vi "LuaVIEW Push (flat data).vi"(0 "flat data":string, 2 "type descriptor":i16[](array[numeric]) format="%x", 5 "LuaVIEW reference in":T1, 7 "include cluster order (false)":bool, 11 "error in (no error)":errorcluster) -> (6 "LuaVIEW reference out":T1, 15 "error out":errorcluster)   [LabVIEW 2013]
doc: "Pushes a Lua-data item onto the stack after translating it from flat LabVIEW data. The most important use for this VI is to transfer compound data from LabVIEW (a cluster or array) to Lua (a table). To perform the translation, this function requires the type descriptor of the LabVIEW type/cluster/array that specifies how the translation is to take place. The translation is recursive and thus handles nested clusters and arrays. If no translation is possible, e.g. because cluster elements are not named, an error is returned. The LuaVIEW manual details which translations are supported. This VI is part of a polymorphic set that supports pushing various data types. To change the type being pushed, pop up on this VI's diagram icon and use the \"Select Type\" sub menu."
uses:
  typedefs/t_LuaVIEW Reference.ctl
  typedefs/et_LuaVIEW CIN Actions.ctl
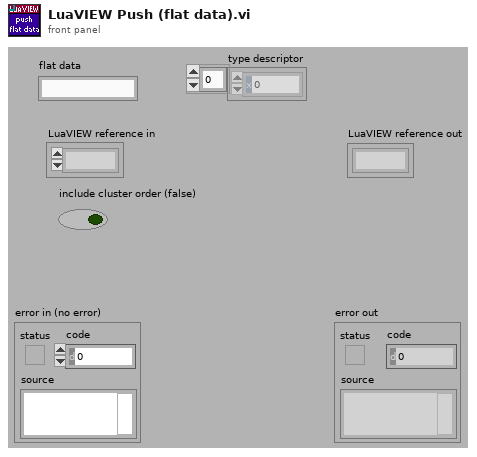
[diagram p1: front panel]
types:
  T1 = typedef "t_LuaVIEW Reference.ctl" = refnum<k1>
  T2 = typedef "et_LuaVIEW CIN Actions.ctl" = enum16{"checksynopsis", "_open", "_registerpublic", "_registerexport", "__never_an_error_result_ns", "luaversion", "cinversion", "_totals", "_taskcount", "pathological", "_unregnextpublic", "registryusecount", "__per_state_actions", "regsetprivate", "regsetindex", "regsetmodule", "_revokeexports", "_usepublic", "prepare", "compile", "execute", "call", "unregstaterefs", "_close", "pullboolean", "pullnumber", "pullI8", "pullU8", "pullI16", "pullU16", "pullI32", "pullU32", "pullobject", "pullrefnum", "pullstring", "pullflat", "pushflat", "pushobject", "getattribute", "setattribute", "stacktostring", "_startyieldtest", "_endyieldtest", "_pollprintbuffer", "__never_an_error_result_ps", "_pollexport", "setclone", "forcecleanup", "gettop", "clearstack", "insert", "pushboolean", "pushnumber", "pushrefnum", "pushstring", "pushnil", "pushvalue", "gettaskref", "settaskref"}
  T3 = typedef "et_LuaVIEW CIN Results.ctl" = enum16{"OK", "error", "main", "call", "clonecall", "modulecall", "exportcall", "index", "yield"}
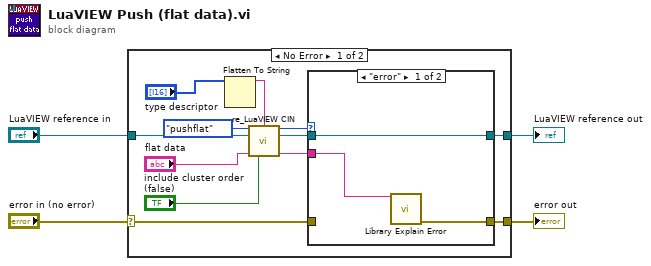
[diagram p0: block diagram]
diagram:
  n1 = case shown="No Error" "error in (no error)" {
    selector: "error in (no error)" -> [w9 w23]
    tunnel: [w13 w22] -> w4
    tunnel: [w11 w23] -> w3
    tunnel: "LuaVIEW reference in" -> [w15 w22]
    frame No Error {
      n2 = Flatten To String(anything="type descriptor") -> (data string=w6:string)  [unwired: 3 in, 2 out]
      n3 = call "re_LuaVIEW CIN.vi"("action"=et_LuaVIEW_CIN_Actions."pushflat", "supplement"=w6, "LuaVIEW reference in"=w15, "string in"="flat data", "boolean in"="include cluster order (false)") -> ("result"=w12:T3, "LuaVIEW reference out"=w14:T1, "string out"=w10:string)  [unwired: 4 in, 4 out]
      n4 = case shown="\"error\"" w12 {
        tunnel: w14 -> [w17 w20]
        tunnel: [w17 w20] -> w13
        tunnel: [w19 w21] -> w11
        tunnel: w10 -> [w18 _]
        tunnel: w9 -> [_ w21]
        frame "error" {
          n5 = call "Library Explain Error.vi"("explanation prefix (none)"=w18) -> ("explained error"=w19:errorcluster)  [unwired: 14 in]
        }
        frame Default {
        }
      }
    }
    frame Error {
    }
  }
  "LuaVIEW reference out" <- w4
  "error out" <- w3
